vi "Reverse Sort Test.vi"(8 "Error In":errorcluster) -> (0 "Error Out":errorcluster)   [LabVIEW 2019, in "Test.lvlib"]
doc: "The VI is a test file that tests the functionality of the reverse sort."
uses:
  Test.lvlib
  <vilib>/addons/_JKI Toolkits/Caraya/classes/Test/Test.lvclass
  <vilib>/addons/_JKI Toolkits/Caraya/classes/Assert/Assert.lvclass
  File Path Operations/File and Path Operations.lvlib
  <vilib>/addons/_JKI Toolkits/Caraya/classes/Assert/Assert Equal Value_Variant.vi
panel:
  # "REVERSE ALPHABETICAL SORT TEST"
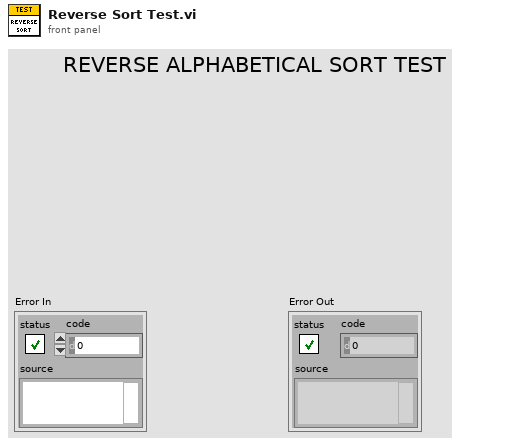
[diagram p1: front panel]
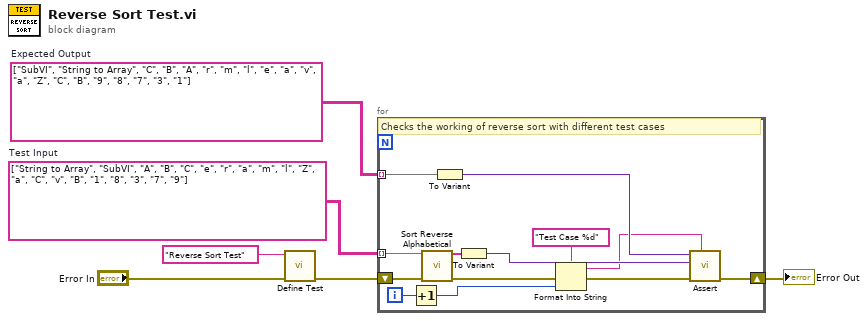
[diagram p0: block diagram]
diagram:
  w1 = string[][] [["SubVI", "String to Array", "C", "B", "A"], ["r", "m", "l", "e", "a"], ["v", "a", "Z", "C", "B"], ["9", "8", "7", "3", "1"]]  # Expected Output
  w2 = string[][] [["String to Array", "SubVI", "A", "B", "C"], ["e", "r", "a", "m", "l"], ["Z", "a", "C", "v", "B"], ["1", "8", "3", "7", "9"]]  # Test Input
  n1 = call <vilib>:"Define Test.vi"("error in (no error)"="Error In", "Label (VI Title)"="Reverse Sort Test") -> ("error out"=w4:errorcluster)  [unwired: 8 in, 1 out]
  n2 = for {
    tunnel: w2 -> [w17] mode=indexing
    shift-right: [w16] -> w3
    shift-left: w4 -> [w19]
    tunnel: w1 -> [w13] mode=indexing
    i -> [w10]
    # "Checks the working of reverse sort with different test cases"
    n3 = Increment(x=w10) -> (x+1=w9:i32)
    n4 = call "Sort Reverse Alphabetical.vi"("Unsorted Array"=w17, "Error In"=w19) -> ("Sorted Array"=w15:string[], "Error Out"=w18:errorcluster)  [unwired: 12 in]
    n5 = To Variant(anything=w13) -> (Variant=w12:variant)
    n6 = To Variant(anything=w15) -> (Variant=w14:variant)
    n7 = Format Into String(format string="Test Case %d", error in=w18, w9) -> (resulting string=w7:string, error out=w11:errorcluster)  [unwired: 1 in]
    n8 = call-poly <vilib>:"Assert.vi"("Label"=w7, "error in (no error)"=w11, "Y"=w14, "X"=w12) -> ("error out"=w16:errorcluster)  [unwired: 6 in, 1 out]
  }
  "Error Out" <- w3
